vi "SGUI Get Boolean State By Label.vi"(7 "generate error if not found? (True)":bool=TRUE, 10 "error in":errorcluster, 11 "control label ('btn stop')":string="btn stop") -> (2 "error out":errorcluster, 3 "binary state out":bool, 5 "found and type matches?":bool)   [LabVIEW 2020, in "varilib.lvlib"]
doc: "Reads state of boolean control pointed by its label. The reference and label must be first registered by calling 'SGUI Register Controls'. If not found or not a boolean, it will by default return error however it ignores input error (executes anyway)."
uses:
  varilib.lvlib
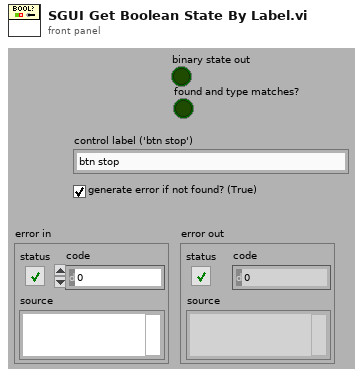
[diagram p1: front panel]
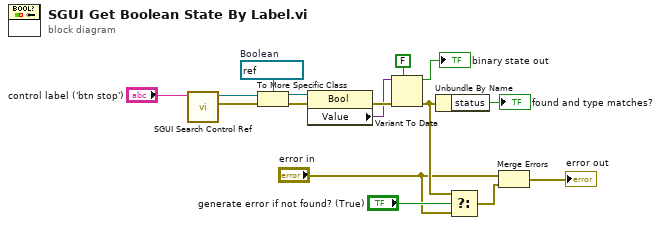
[diagram p0: block diagram]
diagram:
  w12 = refnum<vi> refnum  # Boolean
  n1 = call "SGUI Search Control Ref.vi"("control label (empty)"="control label ('btn stop')") -> ("error out"=w16:errorcluster, "control ref out"=w15:refnum<vi>)  [unwired: 8 in, 1 out]
  n2 = To More Specific Class(target class=w12, reference=w15, error in=w16) -> (specific class reference=w13:refnum<vi>, error out=w14:errorcluster)
  n3 = property class="Bool"(reference=w13, error in=w14) -> (error out=w11:errorcluster, "Value"=w10:variant)  [unwired: 1 out]
  n4 = Variant To Data(error in=w11, type=FALSE, Variant=w10) -> (data=→"binary state out":bool, error out=w2:errorcluster)
  n5 = Unbundle By Name(w2) -> ("status"=→"found and type matches?":bool)
  n6 = Select(t=w2, s="generate error if not found? (True)", f="error in") -> (s? t:f=w4:errorcluster)
  n7 = Merge Errors("error in", w4) -> (→"error out":errorcluster)
